vi "Update P.vi"(8 "error in (no error)":errorcluster, 10 "SLAM In":T3, 11 "New LM's In":T2(array[cluster])) -> (0 "error out":errorcluster, 2 "SLAM Out":T3, 3 "New LM's Out":T2(array[cluster]))   [LabVIEW 2009]
uses:
  <vilib>/Analysis/Matrix/Datatypes/RealMatrix.ctl
  Controls/SLAM.ctl
  <vilib>/Analysis/Matrix/NI_Matrix.lvlib
panel:
  out "ID":dbl
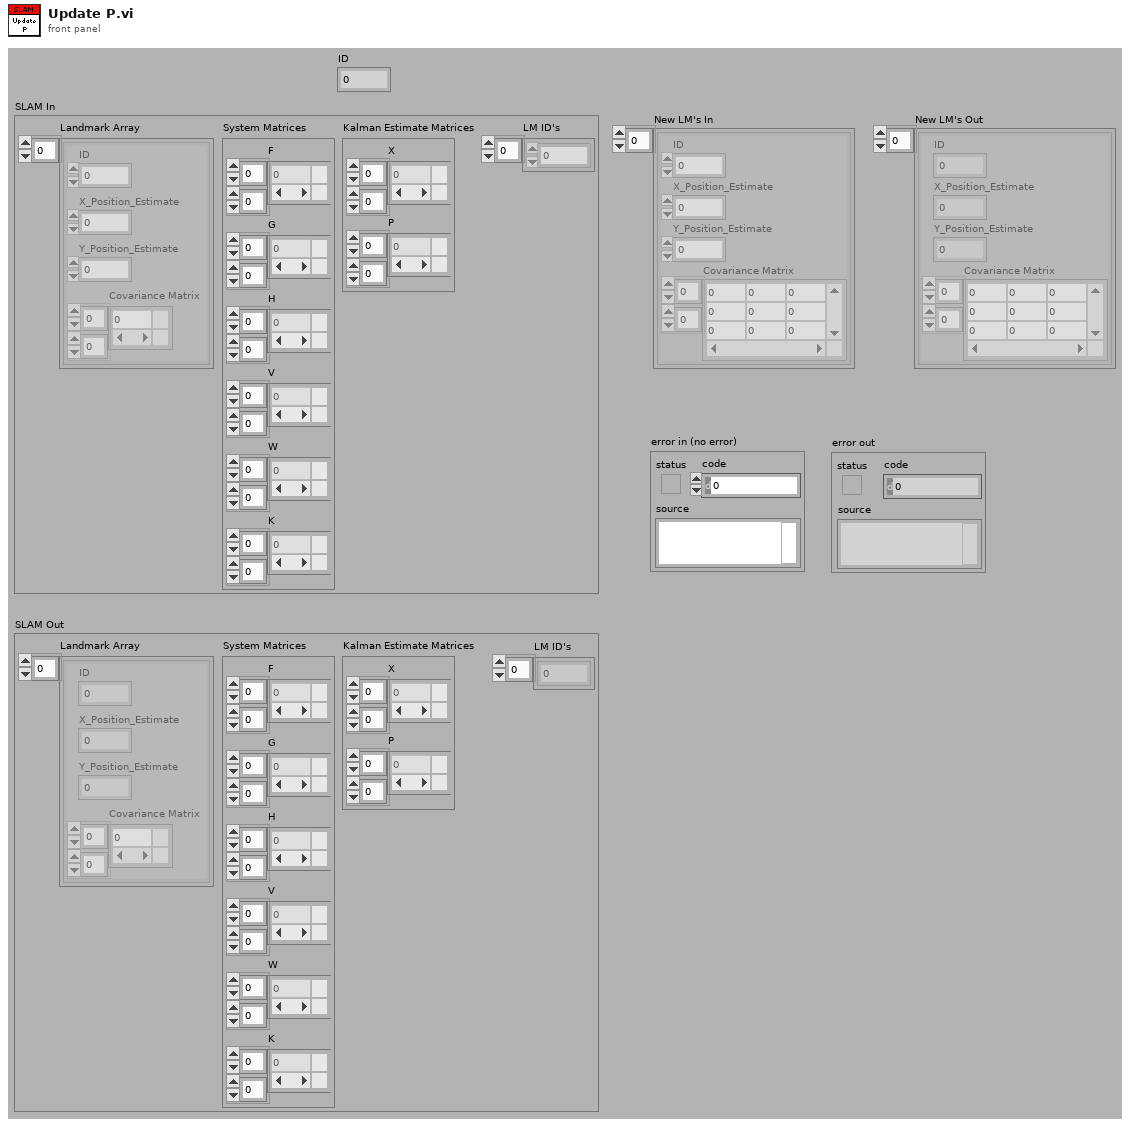
[diagram p1: front panel]
types:
  T1 = typedef "NI_Matrix.lvlib/RealMatrix.ctl" = dbl[][]
  T2 = cluster{"ID":dbl, "X_Position_Estimate":dbl, "Y_Position_Estimate":dbl, "Covariance Matrix":T1}[]
  T3 = typedef "SLAM.ctl" = cluster{"Landmark Array":cluster{"ID":dbl, "X_Position_Estimate":dbl, "Y_Position_Estimate":dbl, "Covariance Matrix":T1}[], "System Matrices":cluster{"F":T1, "G":T1, "H":T1, "V":T1, "W":T1, "K":T1}, "Kalman Estimate Matrices":cluster{"X":T1, "P":T1}, "LM ID's":dbl[]}
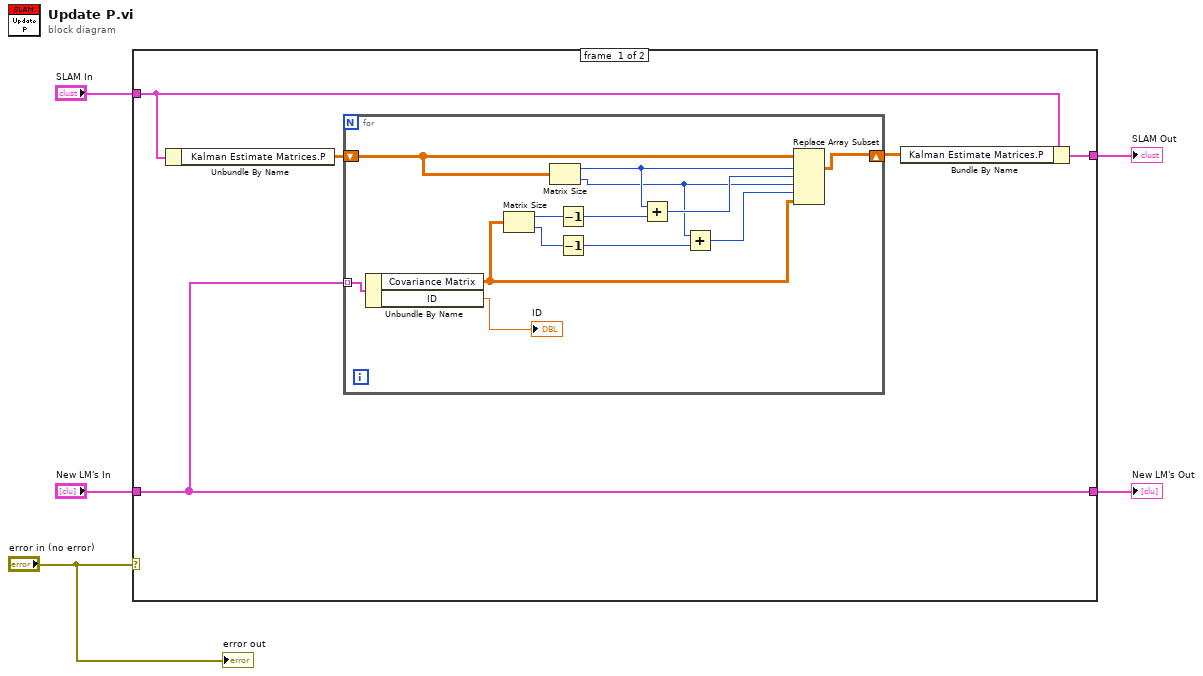
[diagram p0: block diagram]
diagram:
  n1 = case shown="No Error" "error in (no error)" {
    tunnel: "SLAM In" -> [w10 w24]
    tunnel: "New LM's In" -> [w6 w25]
    tunnel: [w9 w24] -> w3
    tunnel: [w6 w25] -> w2
    frame #0 {
      n2 = Unbundle By Name(w10) -> ("Kalman Estimate Matrices.P"=w7:T1)
      n3 = for {
        shift-right: [w18] -> w8
        shift-left: w7 -> [w17]
        tunnel: w6 -> [w16] mode=indexing
        n4 = Unbundle By Name(w16) -> ("Covariance Matrix"=w12:T1, "ID"=→"ID":dbl)
        n5 = Matrix Size(0:w12) -> (1:w15:i32, 2:w14:i32)
        n6 = Matrix Size(0:w17) -> (1:w23:i32, 2:w21:i32)
        n7 = Decrement(x=w15) -> (x-1=w19:i32)
        n8 = Decrement(x=w14) -> (x-1=w13:i32)
        n9 = Add(x=w23, y=w19) -> (x+y=w22:i32)
        n10 = Add(x=w21, y=w13) -> (x+y=w20:i32)
        n11 = Replace Array Subset(array=w17, new element=w12, index (dim 0)=w23, index (dim 1)=w22, index (dim 2)=w21, index (dim 3)=w20) -> (w18:T1)
      }
      n12 = Bundle By Name(cluster=w10, "Kalman Estimate Matrices.P"=w8) -> (w9:T3)
    }
    frame #1 {
    }
  }
  "New LM's Out" <- w2
  "SLAM Out" <- w3
  "error out" <- "error in (no error)"
